vi "Automatic_electromotor.vi"() -> ()   [LabVIEW 2010]
panel:
  in  "?":i8(slide) step=1 scale=0.0..4.0
  out "?":dbl
  in  "stop":bool
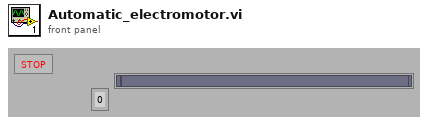
[diagram p1: front panel]
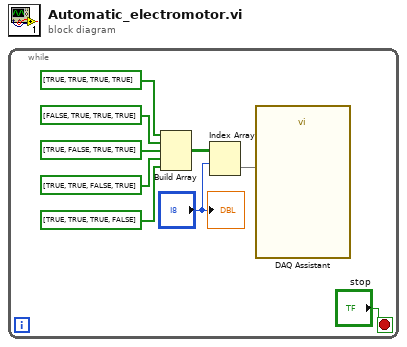
[diagram p0: block diagram]
diagram:
  n1 = while {
    stop <- "stop" stop-if-true
    n2 = Build Array(bool[] [TRUE, TRUE, TRUE, TRUE], bool[] [FALSE, TRUE, TRUE, TRUE], bool[] [TRUE, FALSE, TRUE, TRUE], bool[] [TRUE, TRUE, FALSE, TRUE], bool[] [TRUE, TRUE, TRUE, FALSE]) -> (w8:bool[][])
    n3 = Index Array(array=w8, index (row)="?") -> (element=w3:bool[])  [unwired: 1 in]
    n4 = call "DAQ Assistant"("data"=w3) -> ()  [unwired: 17 in, 2 out]
    "?" <- "?"
  }
